vi "Call Send Cal Cmd.vi"(2 "error in":errorcluster, 3 "VISA resource name":refnum<visa-resource-name>) -> (0 "error out":errorcluster, 1 "VISA resource name out":refnum<visa-resource-name>)   [LabVIEW 2012]
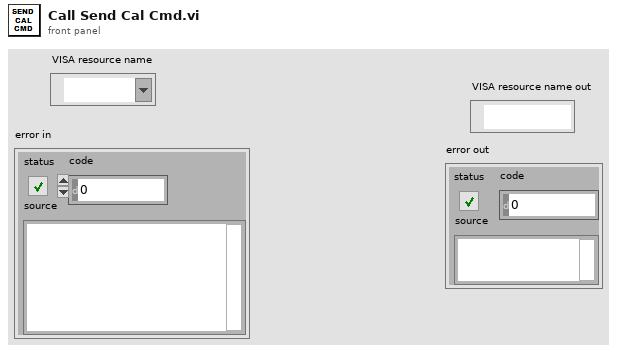
[diagram p1: front panel]
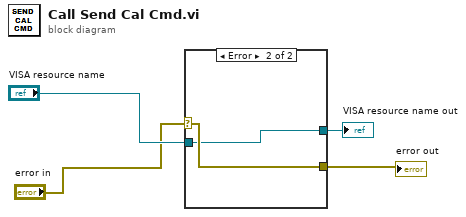
[diagram p0: block diagram]
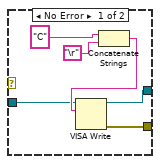
[diagram p2: hidden frame]
diagram:
  n1 = case shown="Error" "error in" {
    selector: "error in" -> [_ w12]
    tunnel: "VISA resource name" -> [w7 w11]
    tunnel: [w6 w12] -> w3
    tunnel: [w5 w11] -> w2
    frame No Error {
      n2 = Concatenate Strings("C" ("string"), "\r") -> (w10:string)
      n3 = VISA Write(VISA resource name=w7, write buffer=w10) -> (VISA resource name out=w5:refnum<visa-resource-name>, error out=w6:errorcluster)  [unwired: 1 in, 1 out]
    }
    frame Error {
    }
  }
  "error out" <- w3
  "VISA resource name out" <- w2
